vi "MFCclient.vi"() -> ()   [LabVIEW 2016]
panel:
  in  "String":string
  in  "Valve":bool
  in  "Setpoint":dbl(slide) max=100.0 step=10.0 scale=0.0..100.0
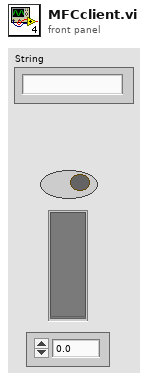
[diagram p1: front panel]
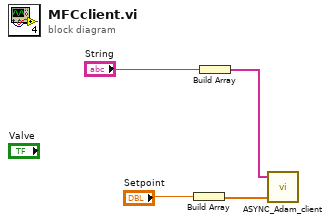
[diagram p0: block diagram]
diagram:
  n1 = Build Array("Setpoint") -> (w4:dbl[])
  n2 = Build Array("String") -> (w2:string[])
  n3 = call "ASYNC_Adam_client.vi"("Values"=w4, "Channel Names"=w2) -> ()  [unwired: 1 in, 2 out]
